vi "Dpc Set Pin Direction.vi"(7 "ptrid":u16, 8 "error in (no error)":errorcluster, 9 "perc":i32, 10 "fsDir":u32, 11 "hif":u32) -> (0 "error out":errorcluster, 1 "perc out":i32, 2 "function return":i32, 3 "hif out":u32, 5 "ptrid out":u16)   [LabVIEW 2011, in "LVH-Adept.lvlib" / "DPCUTIL.lvlib"]
doc: "DPCAPI BOOL DpcSetPinDirection(HANDLE hif, DWORD fsDir, ERC * perc, TRID * ptrid);"
uses:
  DPCUTIL.lvlib
  dpcutil.dll
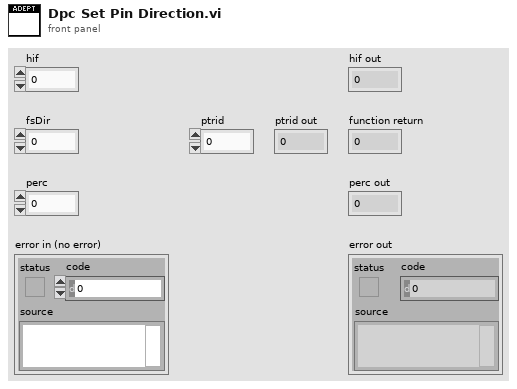
[diagram p1: front panel]
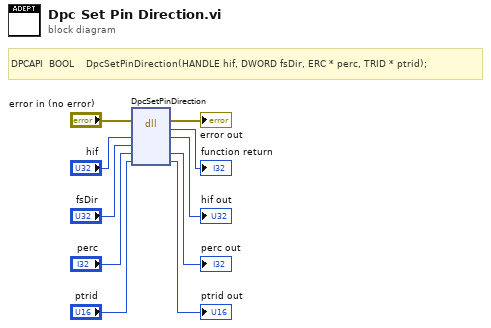
[diagram p0: block diagram]
diagram:
  # "DPCAPI  BOOL    DpcSetPinDirection(HANDLE hif, DWORD fsDir, ERC * perc, TRID * ptrid);"
  n1 = dll-call lib="dpcutil.*" fn="DpcSetPinDirection"(error in="error in (no error)", "hif"="hif", "fsDir"="fsDir", "perc"="perc", "ptrid"="ptrid") -> (error out=→"error out":errorcluster, →"function return":i32, "hif"=→"hif out":u32, "perc"=→"perc out":i32, "ptrid"=→"ptrid out":u16)  [unwired: 3 in, 1 out]
